vi "kD2AChrisBoardTar.vi"(10 "Funny 10 Input":i16[](array[numeric])=[0, 0, 0, 0, 0, 0, 0, 0, 0, 0]) -> (2 "ToFIFO":u16[](array[numeric]))   [LabVIEW 2010, in "kevLib2010.lvlib"]
uses:
  kevLib2010.lvlib
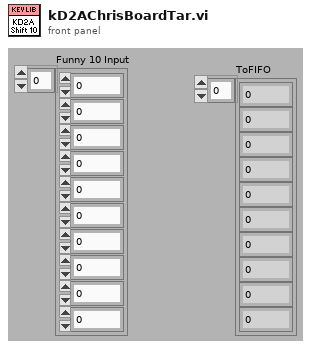
[diagram p1: front panel]
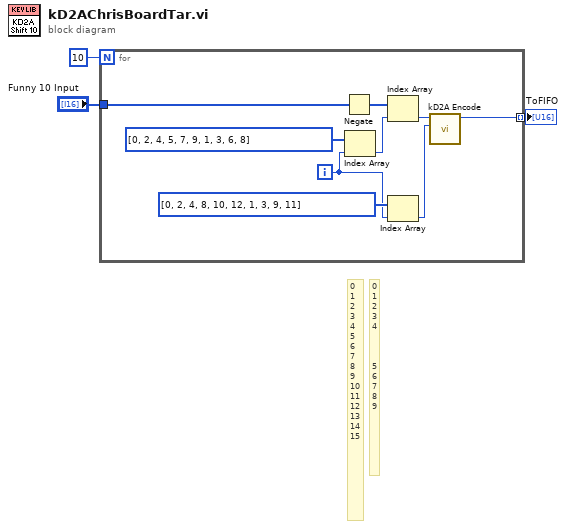
[diagram p0: block diagram]
diagram:
  # "0\n1\n2\n3\n4\n\n\n\n5\n6\n7\n8\n9"
  # "0\n1\n2\n3\n4\n5\n6\n7\n8\n9\n10\n11\n12\n13\n14\n15"
  n1 = for {
    N: 10 -> [_]
    tunnel: "Funny 10 Input" -> [w11]
    tunnel: [w6] -> w1 mode=indexing
    i -> [w9]
    n2 = Negate(x=w11) -> (-x=w5:i16[])
    n3 = Index Array(array=i32[] [0, 2, 4, 5, 7, 9, 1, 3, 6, 8], index=w9) -> (element=w8:i32)
    n4 = Index Array(array=w5, index=w8) -> (element=w7:i16)
    n5 = Index Array(array=u8[] [0, 2, 4, 8, 10, 12, 1, 3, 9, 11], index=w9) -> (element=w4:u8)
    n6 = call "kD2A Encode.vi"("Position"=w4, "Value"=w7) -> ("Coded Output"=w6:u16)  [unwired: 9 in]
  }
  "ToFIFO" <- w1
